vi "Single_meas.vi"(9 "Step Bias [V]":ext=5.0, 10 "Stop Bias [V]":ext=40.0, 11 "Start Bias [V]":ext) -> (3 "Array":ext[](array[numeric]))   [LabVIEW 2017]
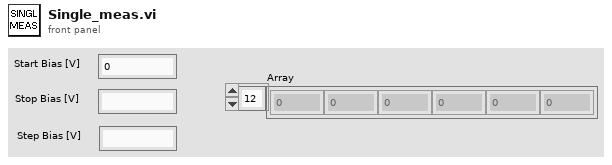
[diagram p1: front panel]
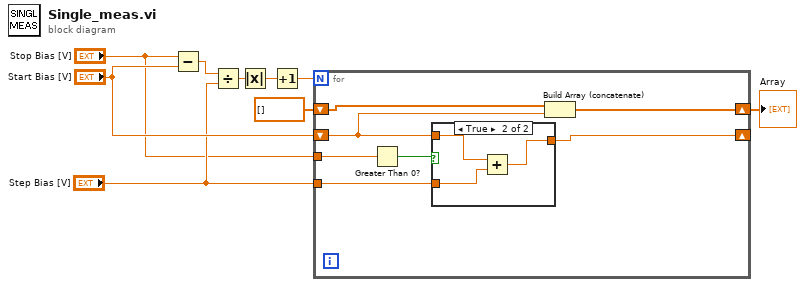
[diagram p0: block diagram]
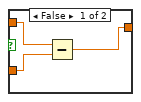
[diagram p2: hidden frame]
diagram:
  n1 = Subtract(x="Stop Bias [V]", y="Start Bias [V]") -> (x-y=w8:ext)
  n2 = Divide(x=w8, y="Step Bias [V]") -> (x/y=w9:ext)
  n3 = Absolute Value(x=w9) -> (abs(x)=w7:ext)
  n4 = Increment(x=w7) -> (x+1=w6:ext)
  n5 = for {
    N: w6 -> [_]
    tunnel: "Step Bias [V]" -> [w16]
    shift-right: [w15] -> _
    shift-left: "Start Bias [V]" -> [w12]
    shift-right: [w14] -> w2
    shift-left: ext[] [] -> [w13]
    tunnel: "Stop Bias [V]" -> [w10]
    n6 = Greater Than 0?(x=w10) -> (x > 0?=w11:bool)
    n7 = case shown="True" w11 {
      tunnel: w16 -> [w18 w22]
      tunnel: [w17 w21] -> w15
      tunnel: w12 -> [w19 w20]
      frame False {
        n8 = Subtract(x=w19, y=w18) -> (x-y=w17:ext)
      }
      frame True {
        n9 = Add(x=w20, y=w22) -> (x+y=w21:ext)
      }
    }
    n10 = Build Array (concatenate)(w13, w12) -> (w14:ext[])
  }
  "Array" <- w2
